vi "UpdateSettingsClusterByName.vi"(8 "error in (no error)":errorcluster, 9 "ElementValue":variant, 10 "ElementLabel":string, 11 "Picomotor8742 in":refnum<class "Picomotor8742.lvclass">) -> (0 "error out":errorcluster, 2 "Success?":bool, 3 "Picomotor8742 out":refnum<class "Picomotor8742.lvclass">)   [LabVIEW 2013, in "Picomotor8742.lvclass"]
uses:
  Picomotor8742.lvclass
  Picomotor8742.lvclass/Picomotor8742.ctl
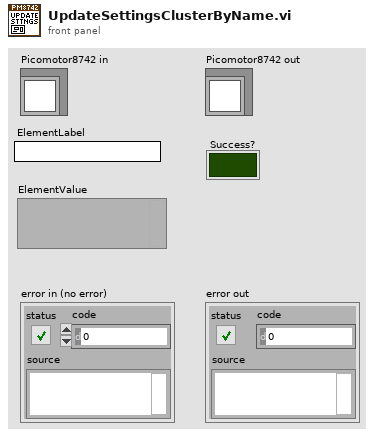
[diagram p1: front panel]
types:
  T1 = typedef "Picomotor8742.lvclass/SettingsTypdef.ctl" = cluster{"Position":cluster{"device 1":cluster{"Value":dbl, "Min":dbl, "Max":dbl, "StepSize":dbl, "Tolerance":dbl, "ValueActual":dbl}, "device 2":cluster{"Value":dbl, "Min":dbl, "Max":dbl, "StepSize":dbl, "Tolerance":dbl, "ValueActual":dbl}, "device 3":cluster{"Value":dbl, "Min":dbl, "Max":dbl, "StepSize":dbl, "Tolerance":dbl, "ValueActual":dbl}, "device 4":cluster{"Value":dbl, "Min":dbl, "Max":dbl, "StepSize":dbl, "Tolerance":dbl, "ValueActual":dbl}}, "ipaddress":string, "StepSize":cluster{"device 1":cluster{"Value":dbl, "Min":dbl, "Max":dbl, "StepSize":dbl, "Tolerance":dbl, "ValueActual":dbl}, "device 2":cluster{"Value":dbl, "Min":dbl, "Max":dbl, "StepSize":dbl, "Tolerance":dbl, "ValueActual":dbl}, "device 3":cluster{"Value":dbl, "Min":dbl, "Max":dbl, "StepSize":dbl, "Tolerance":dbl, "ValueActual":dbl}, "device 4":cluster{"Value":dbl, "Min":dbl, "Max":dbl, "StepSize":dbl, "Tolerance":dbl, "ValueActual":dbl}}, "relativeMove":cluster{"device 1neg":T2, "device 2neg":T2, "device 3neg":T2, "device 1pos":T2, "device 2pos":T2, "device 3pos":T2, "device 4neg":T2, "device 4pos":T2}}
  T2 = typedef "OnOffTypeDef.ctl" = enum16{"off", "on"}
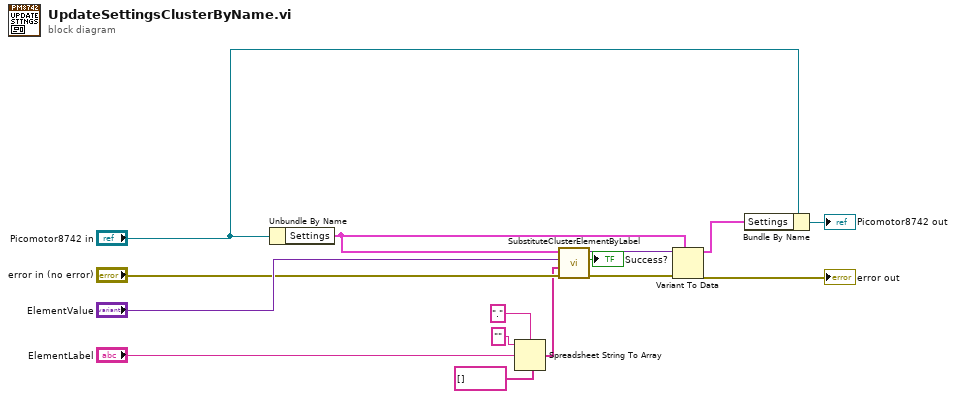
[diagram p0: block diagram]
diagram:
  n1 = Unbundle By Name("Picomotor8742 in") -> ("Settings"=w12:T1)
  n2 = Spreadsheet String To Array(delimiter (Tab)=".", format string="", spreadsheet string="ElementLabel", array type (2D Dbl)=string[] []) -> (array=w3:string[])
  n3 = call "SubstituteClusterElementByLabel.vi"("error in (no error)"="error in (no error)", "ElementHierarchy"=w3, "NewElementValue"="ElementValue", "ClusterIn"=w12) -> ("ErrorOut"=w10:errorcluster, "Success?"=→"Success?":bool, "UpdatedClusterOut"=w11:variant)  [unwired: 5 in]
  n4 = Variant To Data(error in=w10, type=w12, Variant=w11) -> (data=w14:T1, error out=→"error out":errorcluster)
  n5 = Bundle By Name(cluster="Picomotor8742 in", "Settings"=w14) -> (→"Picomotor8742 out":refnum<class "Picomotor8742.lvclass">)
